vi "SENS_CORR_COLL_METH.vi"(0 "VISA IN":refnum<visa-resource-name>, 1 "Method":string, 5 "error in":errorcluster, 7 "Channel":i32) -> (14 "VISA Out":refnum<visa-resource-name>, 19 "error out":errorcluster)   [LabVIEW 2018, in "PNA-X.lvlib"]
doc: "SENSe<cnum>:CORRection:COLLect:METHod <char> \n(Read-Write) For UNGUIDED calibration, sets the calibration method (also known as 'Calibration \nType' on calibration dialog box.) To select a Cal Type from a Cal Set, use CALC:CORR:TYPE. \nNote: Before using this command you must select a measurement using CALC:PAR:SEL. You can \nselect one measurement for each channel. \nParameters \n<cnum> Any existing channel number. If unspecified, value is set to 1 \n<char> Choose from: \nMethod Description \nNONE No Cal method \nREFL1OPEN Response Open \nREFL1SHORT or \nREFL1 \nResponse Short \nREFL3 Full 1 port \nRPOWer Receiver Power Cal \nTRAN1 Response Thru \nTRAN2 Response Thru and Isolation \nSPARSOLT Full SOLT 2 port \nSPARTRL TRL Cal (not available on all PNAs.) \nExamples SENS:CORR:COLL:METH REFL1 \nsense2:correction:collect:method sparsolt \nQuery Syntax SENSe<cnum>:CORRection:COLLect:METHod? \nReturn Type Character \nDefault Not Applicable"
uses:
  PNA-X.lvlib
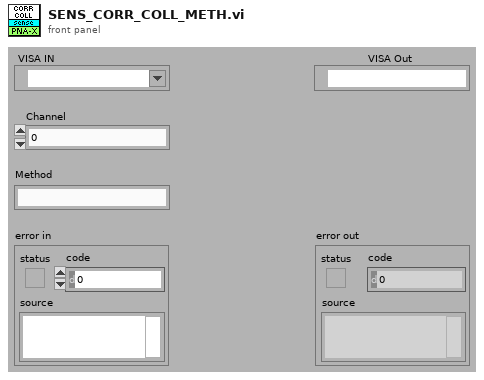
[diagram p1: front panel]
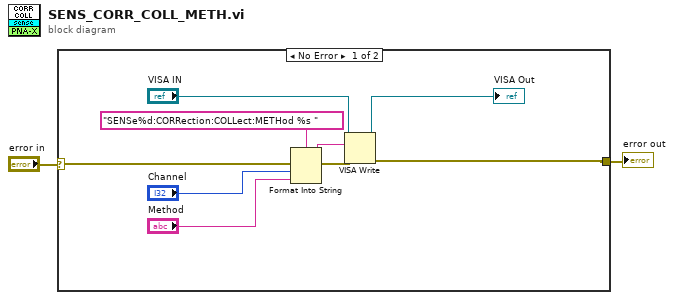
[diagram p0: block diagram]
diagram:
  n1 = case shown="No Error" "error in" {
    selector: "error in" -> [w11 w12]
    tunnel: [w6 w12] -> w1
    frame No Error {
      n2 = Format Into String(format string="SENSe%d:CORRection:COLLect:METHod %s " ("Cmdline"), error in=w11, "Channel", "Method") -> (resulting string=w9:string, error out=w10:errorcluster)  [unwired: 1 in]
      n3 = VISA Write(VISA resource name="VISA IN", write buffer=w9, error in (no error)=w10) -> (VISA resource name out=→"VISA Out":refnum<visa-resource-name>, error out=w6:errorcluster)  [unwired: 1 out]
    }
    frame Error {
    }
  }
  "error out" <- w1
